vi "dif array management.vi"(0 "2D array in":dbl[][](array[numeric]), 1 "col sel":i32, 4 "new element/subarray":dbl) -> (16 "2D array out":dbl[][](array[numeric]), 18 "1D array out":dbl[](array[numeric]))   [LabVIEW 2019]
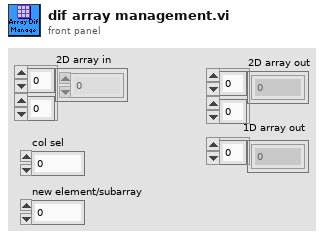
[diagram p1: front panel]
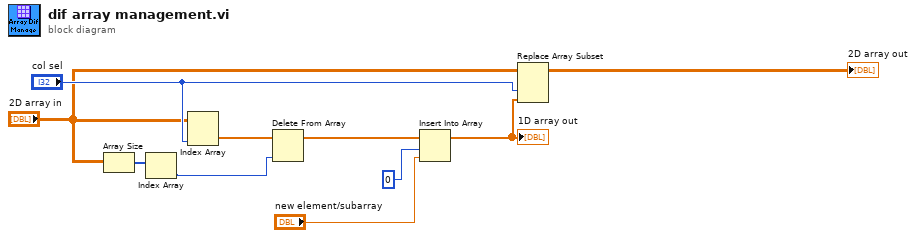
[diagram p0: block diagram]
diagram:
  n1 = Array Size(array="2D array in") -> (size(s)=w2:i32[])
  n2 = Index Array(array=w2) -> (element=w1:i32)  [unwired: 1 in]
  n3 = Index Array "Index Array"(array="2D array in", index (col)="col sel") -> (element=w4:dbl[])  [unwired: 1 in]
  n4 = Delete From Array "Delete From Array"(array=w4, index=w1) -> (array with subset deleted=w9:dbl[])  [unwired: 1 in, 1 out]
  n5 = Insert Into Array "Insert Into Array"(array=w9, index=0, new element="new element/subarray") -> (w8:dbl[])
  "1D array out" <- w8
  n6 = Replace Array Subset "Replace Array Subset"(array="2D array in", new element=w8, index (col)="col sel") -> (→"2D array out":dbl[][])  [unwired: 1 in]
